vi "PeriodicTimer.vi"(6 "Initial":bool, 10 "Reset":bool, 11 "Period (ms)":i32) -> (0 "Iterator":i32, 2 "Square Wave":bool, 3 "Period Expired (one pulse)":bool)   [LabVIEW 2023, in "ArduinoSerialBling.lvlib"]
uses:
  ArduinoSerialBling.lvlib
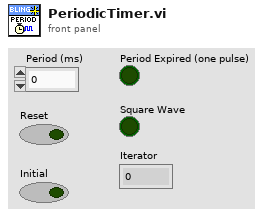
[diagram p1: front panel]
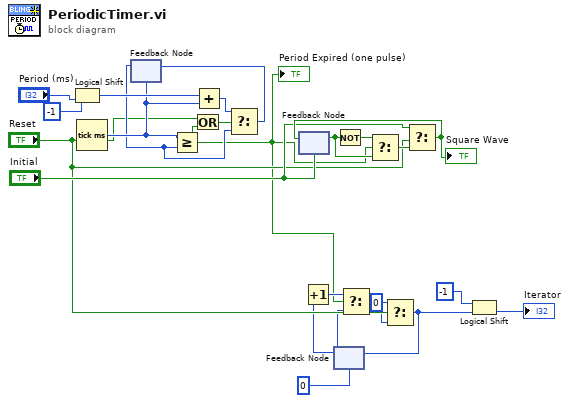
[diagram p0: block diagram]
diagram:
  n1 = Logical Shift(y=i16 -1, x="Period (ms)") -> (x << y=w17:i32)
  n2 = Tick Count (ms)() -> (millisecond timer value=w12:u32)
  n3 = feedback #1(w12) -> (w11:u32)
  n4 = Greater Or Equal?(x=w12, y=w11) -> (x >= y?=w3:bool)
  "Period Expired (one pulse)" <- w3
  n5 = Or(x="Reset", y=w3) -> (x .or. y?=w18:bool)
  n6 = Add(x=w17, y=w12) -> (x+y=w13:u32)
  n7 = Select(t=w13, s=w18, f=w11) -> (s? t:f=w14:u32)
  n8 = feedback-in #1(w14) -> ()
  n9 = feedback #2("Initial") -> (w20:bool)
  n10 = feedback #3(0) -> (w4:i32)
  n11 = Increment(x=w4) -> (x+1=w5:i32)
  n12 = Not(x=w20) -> (.not. x?=w19:bool)
  n13 = Select(t=w5, s=w3, f=w4) -> (s? t:f=w8:i32)
  n14 = Select(t=w19, s=w3, f=w20) -> (s? t:f=w21:bool)
  n15 = Select(t=0, s="Reset", f=w8) -> (s? t:f=w7:i32)
  n16 = feedback-in #3(w7) -> ()
  n17 = Select(t="Initial", s="Reset", f=w21) -> (s? t:f=w23:bool)
  "Square Wave" <- w23
  n18 = feedback-in #2(w23) -> ()
  n19 = Logical Shift(y=i16 -1, x=w7) -> (x << y=→"Iterator":i32)
